vi "mosbus.vi"() -> ()   [LabVIEW 2014]
uses:
  <vilib>/NI/Modbus Library/API/Wrapper/API Main.lvlib
  <vilib>/NI/Modbus Library/API/Wrapper/Create TCP Master.vi
panel:
  in  "stop":bool
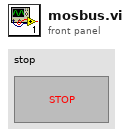
[diagram p1: front panel]
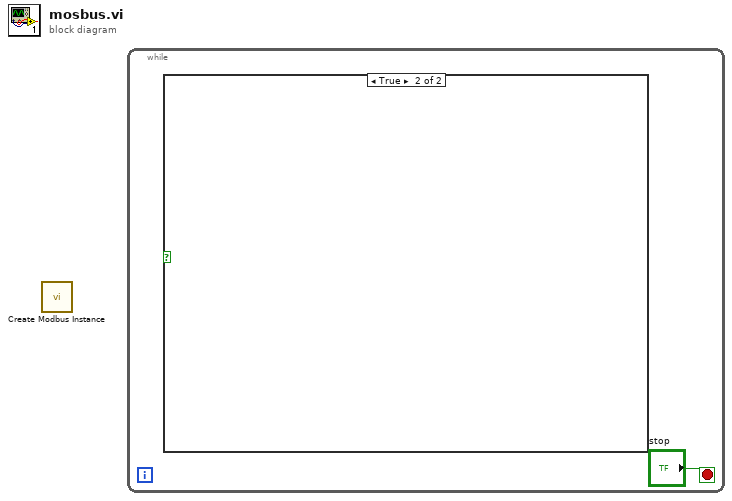
[diagram p0: block diagram]
diagram:
  n1 = call-poly <vilib>:"Create Modbus Instance.vi"() -> ()  [unwired: 10 in, 2 out]
  n2 = while {
    stop <- "stop" stop-if-true
    n3 = case shown="True" {
      selector: _ -> [_ _]
      frame False {
      }
      frame True {
      }
    }
  }
